vi "Save Layout.vi"(8 "error in (no error)":errorcluster, 10 "key":string, 11 "input cluster":T6) -> (0 "error out":errorcluster, 3 "map out":map{string, T1}(c390))   [LabVIEW 2020, in "MDI ViewManager.lvlib"]
uses:
  MDI ViewManager.lvlib
  Typedef/Layout.ctl
  <vilib>/Utility/miscctls.llb/LVPointTypeDef.ctl
  <vilib>/Utility/miscctls.llb/LVBoundsTypeDef.ctl
  <vilib>/Utility/miscctls.llb/LVPositionTypeDef.ctl
  <vilib>/Utility/miscctls.llb/LVRectTypeDef.ctl
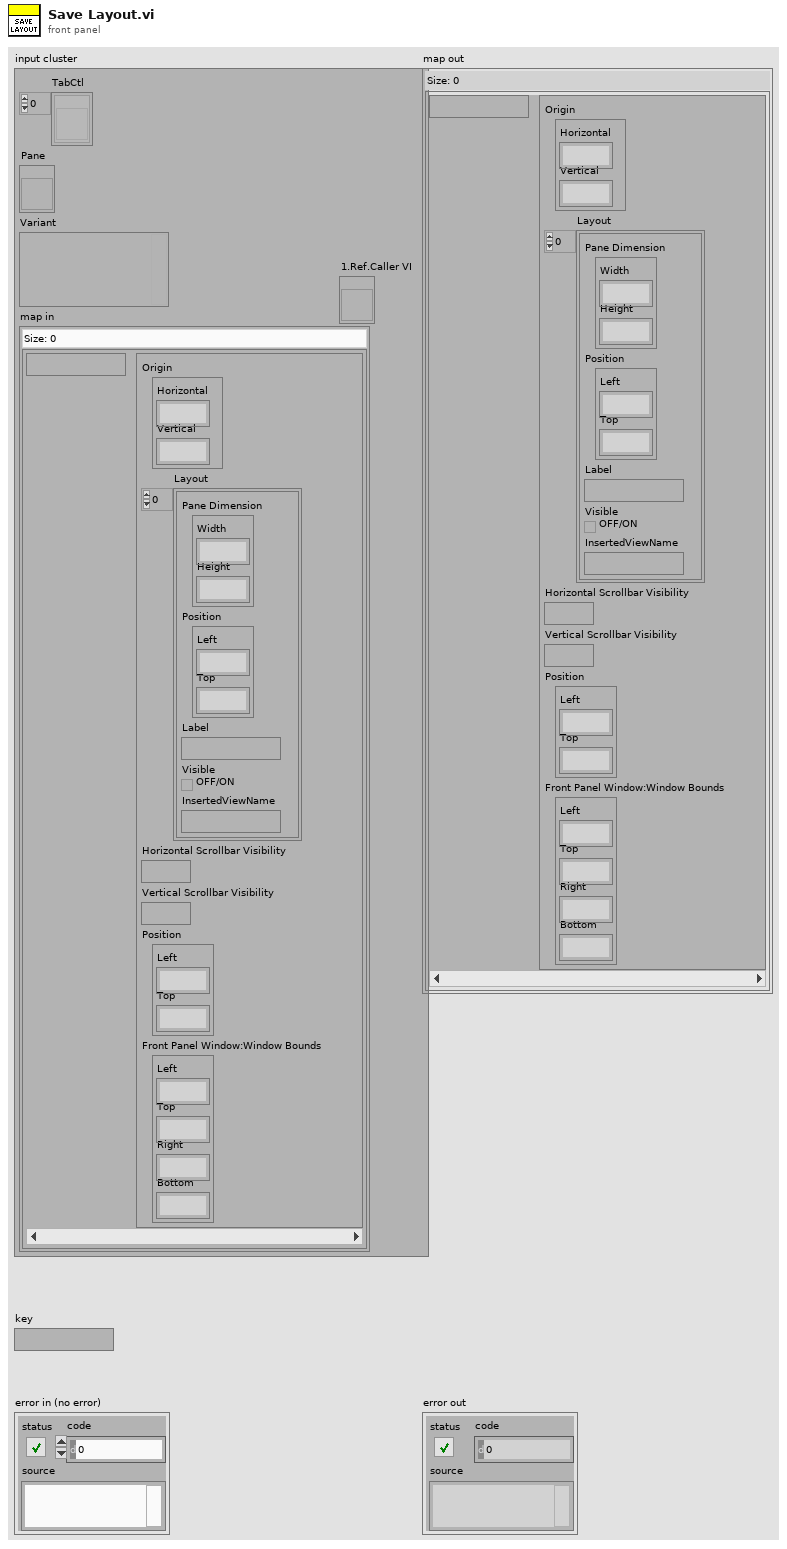
[diagram p1: front panel]
types:
  T1 = typedef "MDI ViewManager.lvlib/Layout.ctl" = cluster{"Origin":T2, "Layout":cluster{"Pane Dimension":T3, "Position":T4, "Label":string, "Visible":bool, "InsertedViewName":string}[], "Horizontal Scrollbar Visibility":enum16{"Always On", "Always Off", "Off While Running"}, "Vertical Scrollbar Visibility":enum16{"Always On", "Always Off", "Off While Running"}, "Position":T4, "Rect":T5}
  T2 = typedef "LVPointTypeDef.ctl" = cluster{"Horizontal":i16, "Vertical":i16}
  T3 = typedef "LVBoundsTypeDef.ctl" = cluster{"Width":u32, "Height":u32}
  T4 = typedef "LVPositionTypeDef.ctl" = cluster{"Left":i32, "Top":i32}
  T5 = typedef "LVRectTypeDef.ctl" = cluster{"Left":i16, "Top":i16, "Right":i16, "Bottom":i16}
  T6 = cluster{"TabCtl":refnum<vi>[], "Pane":refnum<vi>, "Variant":variant, "map in":map{string, T1}, "1.Ref.Caller VI":refnum<vi>}
  T7 = cluster{"Pane Dimension":T3, "Position":T4, "Label":string, "Visible":bool, "InsertedViewName":string}
  T8 = enum16{"Always On", "Always Off", "Off While Running"}
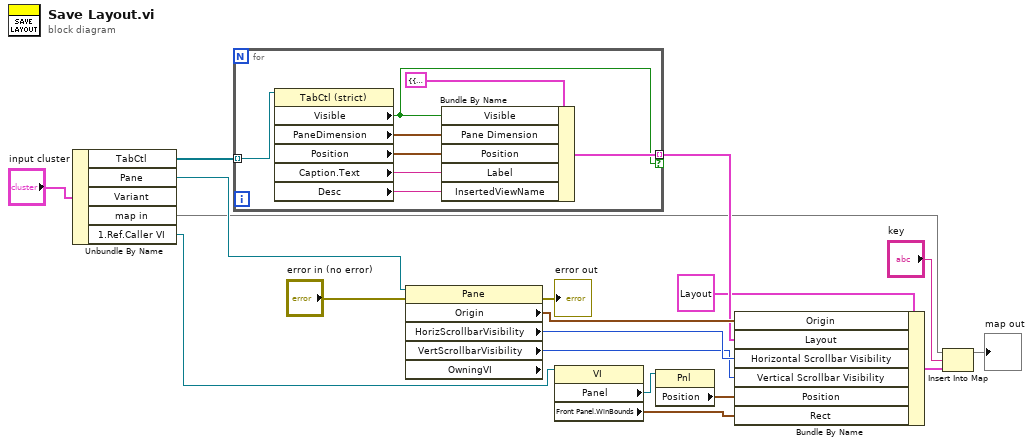
[diagram p0: block diagram]
diagram:
  n1 = Unbundle By Name("input cluster") -> ("TabCtl"=w16:refnum<vi>[], "Pane"=w15:refnum<vi>, "map in"=w11:map{string, T1}, "1.Ref.Caller VI"=w1:refnum<vi>)  [unwired: 1 out]
  n2 = for {
    tunnel: w16 -> [w21] mode=indexing
    tunnel: [w24] -> w17 mode=indexing if=w22
    n3 = property class="TabCtl (strict)"(reference=w21) -> ("Visible"=w22:bool, "PaneDimension"=w26:T3, "Position"=w25:T4, "Caption.Text"=w20:string, "Desc"=w19:string)  [unwired: 1 in, 2 out]
    n4 = Bundle By Name(cluster=T7 {"Pane Dimension"={"Width"=0, "Height"=0}, "Position"={"Left"=0, "Top"=0}, "Label"="", "Visible"=FALSE, "InsertedViewName"=""}, "Visible"=w22, "Pane Dimension"=w26, "Position"=w25, "Label"=w20, "InsertedViewName"=w19) -> (w24:T7)
  }
  n5 = property class="Pane" props=["Origin", "HorizScrollbarVisibility", "VertScrollbarVisibility", "OwningVI"](reference=w15, error in="error in (no error)") -> (error out=→"error out":errorcluster, "Origin"=w18:T2, "HorizScrollbarVisibility"=w6:T8, "VertScrollbarVisibility"=w5:T8)  [unwired: 2 out]
  n6 = property class="VI"(reference=w1) -> ("Panel"=w4:refnum<vi>, "Front Panel.WinBounds"=w2:T5)  [unwired: 1 in, 2 out]
  n7 = property class="Pnl"(reference=w4) -> ("Position"=w3:T4)  [unwired: 1 in, 2 out]
  n8 = Bundle By Name(cluster=T1 {"Origin"={"Horizontal"=0, "Vertical"=0}, "Layout"=[], "Horizontal Scrollbar Visibility"=enum."Always On", "Vertical Scrollbar Visibility"=enum."Always On", "Position"={"Left"=0, "Top"=0}, "Rect"={"Left"=0, "Top"=0, "Right"=0, "Bottom"=0}} ("value"), "Origin"=w18, "Layout"=w17, "Horizontal Scrollbar Visibility"=w6, "Vertical Scrollbar Visibility"=w5, "Position"=w3, "Rect"=w2) -> (w8:T1)
  n9 = Insert Into Map(map in=w11, key="key", value=w8) -> (map out=→"map out":map{string, T1})  [unwired: 2 out]
